vi "CreateFile.vi"(11 "Date/time":string) -> (0 "error out":errorcluster, 2 "Date/Time":string, 3 "Byte Stream File out":refnum<file>)   [LabVIEW 2017]
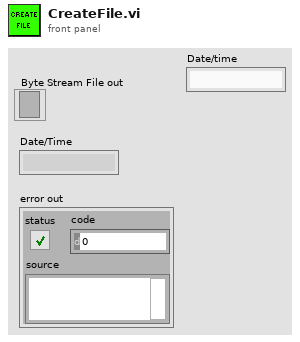
[diagram p1: front panel]
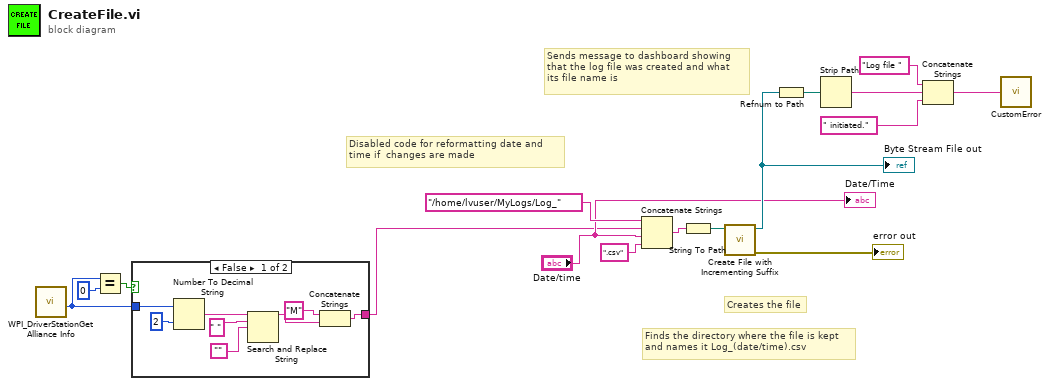
[diagram p0: block diagram]
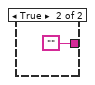
[diagram p2: hidden frame]
diagram:
  # "Finds the directory where the file is kept\nand names it Log_(date/time).csv"
  # "Creates the file"
  # "Sends message to dashboard showing\nthat the log file was created and what \nits file name is"
  # "Disabled code for reformatting date and \ntime if  changes are made"
  n1 = call <vilib>:"WPI_DriverStationGet Alliance Info.vi"() -> ("Match Number"=w5:u16)  [unwired: 6 in, 5 out]
  n2 = Equal?(x=w5, y=u16 0) -> (x = y?=w7:bool)
  n3 = case shown="False" w7 {
    tunnel: [w22 ""] -> w3
    tunnel: w5 -> [w23 _]
    frame False {
      n4 = Number To Decimal String(number=w23, width (-)=i16 2) -> (decimal integer string=w21:string)
      n5 = Search and Replace String(input string=w21, search string=" " ("string"), replace string="") -> (result string=w17:string)  [unwired: 5 in, 3 out]
      n6 = Concatenate Strings("M" ("string"), w17) -> (w22:string)
    }
    frame True {
    }
  }
  n7 = Concatenate Strings("/home/lvuser/MyLogs/Log_" ("string"), w3, "Date/time", ".csv" ("string")) -> (w13:string)
  n8 = String To Path(string=w13) -> (path=w12:path)
  n9 = call <vilib>:"Create File with Incrementing Suffix.vi"("file path"=w12) -> ("error out"=→"error out":errorcluster, "refnum out"=w15:refnum<file>)  [unwired: 8 in, 1 out]
  "Byte Stream File out" <- w15
  n10 = Refnum to Path(1:w15) -> (0:w2:path)
  n11 = Strip Path(path=w2) -> (name=w1:string)  [unwired: 1 out]
  n12 = Concatenate Strings("Log file " ("Source"), w1, " initiated." ("string")) -> (w9:string)
  n13 = call "CustomError.vi"("String"=w9) -> ()  [unwired: 10 in, 1 out]
  "Date/Time" <- "Date/time"
